vi "G#Debugger_NavigateToPreviousTreeItem.vi"(0 "Tree":refnum<vi>, 1 "Tag":string, 5 "error in (no error)":errorcluster) -> (19 "error out":errorcluster)   [LabVIEW 2017, in "G#Debugger.lvlib"]
uses:
  G#Debugger.lvlib
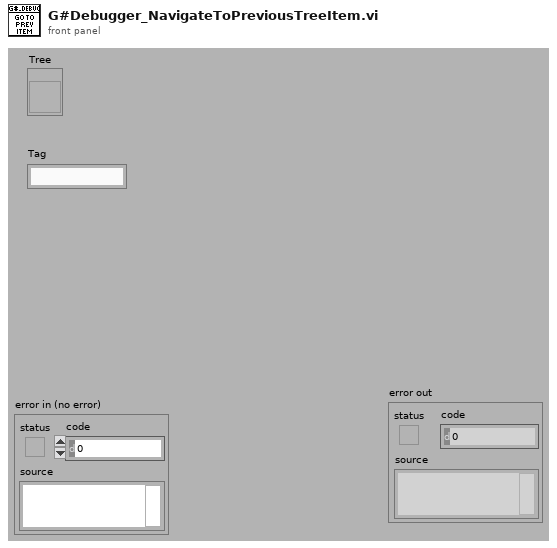
[diagram p1: front panel]
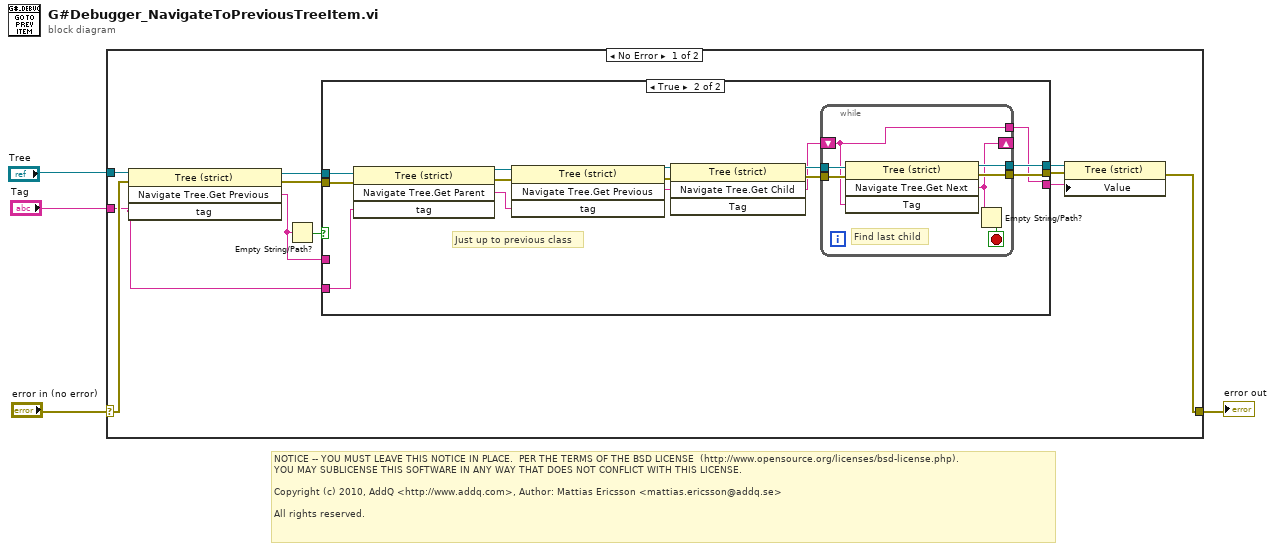
[diagram p0: block diagram]
diagram:
  # "NOTICE -- YOU MUST LEAVE THIS NOTICE IN PLACE.  PER THE TERMS OF THE BSD LICENSE  (http://www.opensource.org/licenses/bsd-license.php).\nYOU MAY SUBLICENSE THIS SOFTWARE IN ANY WAY THAT DOES NOT CONFLICT WITH THIS LICENSE.\n\nCopyright (c) 2010, AddQ <http://www.addq.com>, Author: Mattias Ericsson <mattias.ericsson@addq.se>\n\nAll rights reserved."
  n1 = case shown="No Error" "error in (no error)" {
    selector: "error in (no error)" -> [w13 w41]
    tunnel: [w14 w41] -> w3
    tunnel: "Tag" -> [w5 _]
    tunnel: "Tree" -> [w15 _]
    frame No Error {
      n2 = invoke class="Tree (strict)" method="Navigate Tree.Get Previous"(reference=w15, error in=w13, "tag"=w5) -> (reference out=w7:refnum<vi>, error out=w6:errorcluster, "Navigate Tree:Get Previous"=w8:string)  [unwired: 1 in, 1 out]
      n3 = Empty String/Path?(string/path=w8) -> (empty?=w12:bool)
      n4 = case shown="True" w12 {
        tunnel: w6 -> [w17 w32]
        tunnel: w7 -> [w18 w33]
        tunnel: [w17 w21] -> w11
        tunnel: [w18 w22] -> w10
        tunnel: w8 -> [w16 _]
        tunnel: [w16 w20] -> w9
        tunnel: w5 -> [_ w28]
        frame False {
        }
        frame True {
          # "Just up to previous class"
          n5 = invoke class="Tree (strict)" method="Navigate Tree.Get Parent"(reference=w33, error in=w32, "tag"=w28) -> (reference out=w31:refnum<vi>, error out=w30:errorcluster, "Navigate Tree:Get Parent"=w29:string)  [unwired: 1 in, 1 out]
          n6 = invoke class="Tree (strict)" method="Navigate Tree.Get Previous"(reference=w31, error in=w30, "tag"=w29) -> (reference out=w27:refnum<vi>, error out=w26:errorcluster, "Navigate Tree:Get Previous"=w25:string)  [unwired: 1 in, 1 out]
          n7 = invoke class="Tree (strict)" method="Navigate Tree.Get Child"(reference=w27, error in=w26, "Tag"=w25) -> (reference out=w24:refnum<vi>, error out=w23:errorcluster, "Navigate Tree:Get Child"=w19:string)  [unwired: 1 in, 1 out]
          n8 = while {
            tunnel: w24 -> [w40]
            tunnel: w23 -> [w39]
            tunnel: [w37] -> w22
            tunnel: [w36] -> w21
            shift-right: [w35] -> _
            shift-left: w19 -> [w34]
            tunnel: [w34] -> w20
            stop <- w38 stop-if-true
            # "Find last child"
            n9 = invoke class="Tree (strict)" method="Navigate Tree.Get Next"(reference=w40, error in=w39, "Tag"=w34) -> (reference out=w37:refnum<vi>, error out=w36:errorcluster, "Navigate Tree:Get Next Item"=w35:string)  [unwired: 1 in, 1 out]
            n10 = Empty String/Path?(string/path=w35) -> (empty?=w38:bool)
          }
        }
      }
      n11 = property class="Tree (strict)"(reference=w10, error in=w11, "Value"=w9) -> (error out=w14:errorcluster)  [unwired: 1 out]
    }
    frame Error {
    }
  }
  "error out" <- w3
